vi "GE 5565PIORC.PIO.Read In-Place (1D I8).vi"(5 "count (-1: all)":i32=-1, 8 "error in (no error)":errorcluster, 9 "data in":i8[](array[numeric]), 10 "offset":u32, 11 "GE 5565PIORC in":refnum<class "GE 5565PIORC.lvclass">) -> (0 "error out":errorcluster, 1 "data out":i8[](array[numeric]), 3 "GE 5565PIORC out":refnum<class "GE 5565PIORC.lvclass">)   [LabVIEW 2020, in "GE 5565PIORC.lvclass"]
doc: "Reads <B>count</B> elements of <B>data</B> from the specified <B>offset</B>. The number of elements transferred will be either <B>count</B> or the number of elements in <B>data</B>, whichever is smaller."
uses:
  GE 5565PIORC.lvclass
  <vilib>/Instr/_visa.llb/VISA Register Access Address Space.ctl
  GE 5565PIORC.lvclass/GE 5565PIORC.ctl
  GE 5565PIORC.VISA.Move In-Place.String (U8).vi
  GE 5565PIORC.VISA.Return Handler.vi
  <vilib>/Utility/error.llb/Error Cluster From Error Code.vi
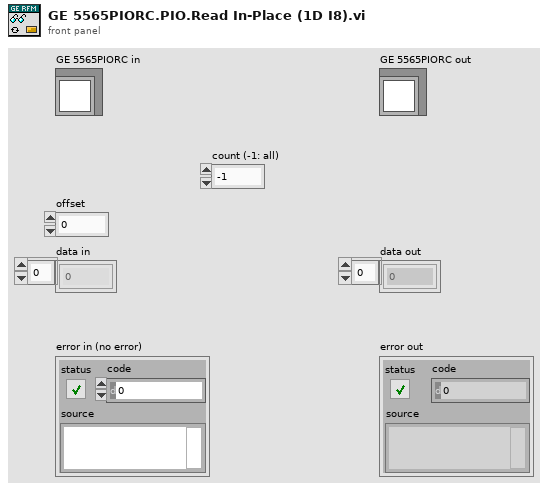
[diagram p1: front panel]
types:
  T1 = typedef "VISA Register Access Address Space.ctl" = u16
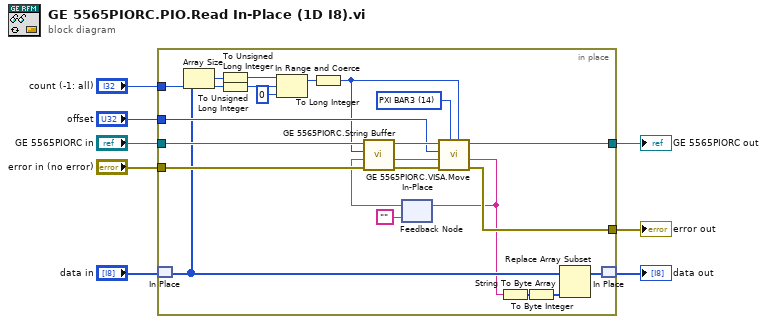
[diagram p0: block diagram]
diagram:
  n1 = in-place {
    in-place-border: "error in (no error)" -> [w24]
    in-place-border: [w12] -> w7
    in-place-border: "GE 5565PIORC in" -> [w25]
    in-place-border: "offset" -> [w17]
    in-place-border: [w27] -> w4
    in-place-border: "count (-1: all)" -> [w19]
    w28 = T1 14 items=["VXI/VME A16"=1, "VXI/VME A24"=2, "VXI/VME A32"=3, "VXI/VME A64"=4, "PXI Memory Allocations"=9, "PXI Configuration"=10, "PXI BAR0"=11, "PXI BAR1"=12, "PXI BAR2"=13, "PXI BAR3"=14, "PXI BAR4"=15, "PXI BAR5"=16] ("address space")
    n2 = in-place-match #1("data in") -> (w16:i8[])
    n3 = Array Size(array=w16) -> (size(s)=w30:i32)
    n4 = To Unsigned Long Integer(number=w30) -> (unsigned 32bit integer=w15:u32)
    n5 = To Unsigned Long Integer(number=w19) -> (unsigned 32bit integer=w14:u32)
    n6 = In Range and Coerce(upper limit=w15, x=w14, lower limit=u32 0) -> (coerced(x)=w18:u32)  [unwired: 1 out]
    n7 = To Long Integer(number=w18) -> (32bit integer=w13:i32)
    n8 = feedback #2("" ("data out")) -> (w21:string)
    n9 = call "GE 5565PIORC.String Buffer.vi"("error in (no error)"=w24, "string buffer in"=w21, "minimum size"=w13, "GE 5565PIORC in"=w25) -> ("error out"=w23:errorcluster, "string buffer out"=w22:string, "GE 5565PIORC out"=w26:refnum<class "GE 5565PIORC.lvclass">)  [unwired: 5 in]
    n10 = call-poly "GE 5565PIORC.VISA.Move In-Place.vi"("count (-1: all)"=w13, "address space"=w28, "error in (no error)"=w23, "data in"=w22, "offset"=w17, "GE 5565PIORC in"=w26) -> ("error out"=w12:errorcluster, "data out"=w11:string, "GE 5565PIORC out"=w27:refnum<class "GE 5565PIORC.lvclass">)  [unwired: 3 in]
    n11 = feedback-in #2(w11) -> ()
    n12 = String To Byte Array(string=w11) -> (unsigned byte array=w10:u8[])
    n13 = To Byte Integer(number=w10) -> (8bit integer=w9:i8[])
    n14 = Replace Array Subset(array=w16, new element=w9) -> (w29:i8[])  [unwired: 1 in]
    n15 = in-place-match #1(w29) -> (→"data out":i8[])
  }
  "GE 5565PIORC out" <- w4
  "error out" <- w7
